vi "Projectile.vi"() -> ()   [LabVIEW 2015]
uses:
  <vilib>/imath/engines/lvmath2/RunTimeEngine/Managers/WorkSpace/UID Generator.vi
  <vilib>/imath/engines/lvmath2/RunTimeEngine/LocalVariableDefStatement/MC_LocalVariableDefStatement_Display.vi
  <vilib>/imath/engines/lvmath2/RunTimeEngine/RunTimeType/NIMS_RunTimeType_From StrictType (excl LVString).vi
  <vilib>/imath/engines/lvmath2/RunTimeEngine/Managers/SymbolTable/Clear UID.vi
  <vilib>/imath/engines/lvmath2/RunTimeEngine/Managers/SymbolTable/NIMS_WorkSpace.lvlib
  <vilib>/imath/engines/lvmath2/RunTimeEngine/NodeEndStatement/NIMS_NodeEndStatement_Output.vi
  <vilib>/imath/engines/lvmath2/RunTimeEngine/ErrorHandling/NIMS_Finalize Error.vi
panel:
  out "XY Graph":cluster{"theta":i32[], "R":dbl[]}(graph)
  in  "Launch Height (m)":dbl
  in  "Launch Speed (m/s)":dbl
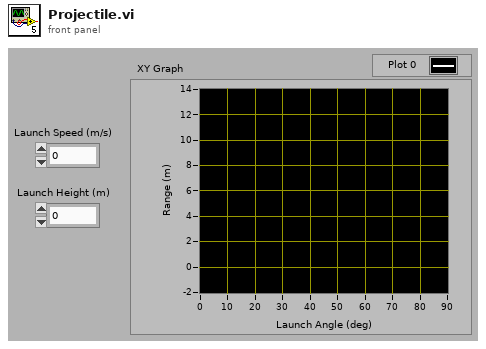
[diagram p1: front panel]
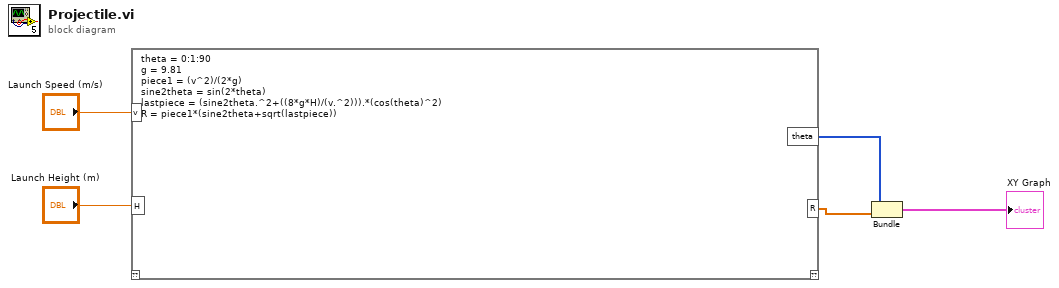
[diagram p0: block diagram]
diagram:
  n1 = mathscript code="theta = 0:1:90\ng = 9.81\npiece1 = (v^2)/(2*g)\nsine2theta = sin(2*theta)\nlastpiece = (sine2theta.^2+((8*g*H)/(v.^2))).*(cos(theta)^2)\nR = piece1*(sine2theta+sqrt(lastpiece))"("v"="Launch Speed (m/s)", "H"="Launch Height (m)") -> ("theta"=w5:i32[], "R"=w1:dbl[])  [unwired: 1 in, 1 out]
  n2 = Bundle("theta"=w5, "R"=w1) -> (→"XY Graph":cluster{"theta":i32[], "R":dbl[]})  [unwired: 1 in]
